vi "Publish Progress Message.vi"(11 "Progress":string) -> ()   [LabVIEW 2023, in "Plugin Generator.lvlib"]
uses:
  Plugin Generator.lvlib
  [Global].vi
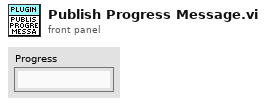
[diagram p1: front panel]
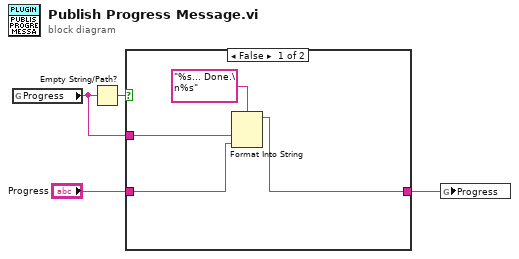
[diagram p0: block diagram]
diagram:
  n1 = global read "[Global].vi" "Progress"() -> (w2:string)
  n2 = Empty String/Path?(string/path=w2) -> (empty?=w4:bool)
  n3 = case shown="False" w4 {
    tunnel: "Progress" -> [w7 w9]
    tunnel: w2 -> [w8 _]
    tunnel: [w5 w9] -> w1
    frame False {
      n4 = Format Into String(format string="%s... Done.\n%s", w8, w7) -> (resulting string=w5:string)  [unwired: 2 in, 1 out]
    }
    frame True {
    }
  }
  n5 = global write "[Global].vi" "Progress"(w1) -> ()
